vi "Read-all-variables.vi"(8 "error in (no error)":errorcluster, 11 "Config. params. ref. in":refnum<data-value>) -> (0 "error out":errorcluster, 2 "Config. vars.":T1, 3 "Config. params. ref.":refnum<data-value>)   [LabVIEW 2013, in "CameraVision.lvlib" / "CV-Configuration.lvclass"]
uses:
  CV-Configuration.lvclass
  Configuration-variables.ctl
  Hardware/Camera/Camera.lvclass
  UI/Module-states.ctl
  CV-Configuration.lvclass/CV-Configuration.ctl
  UI/CV-UI.lvclass
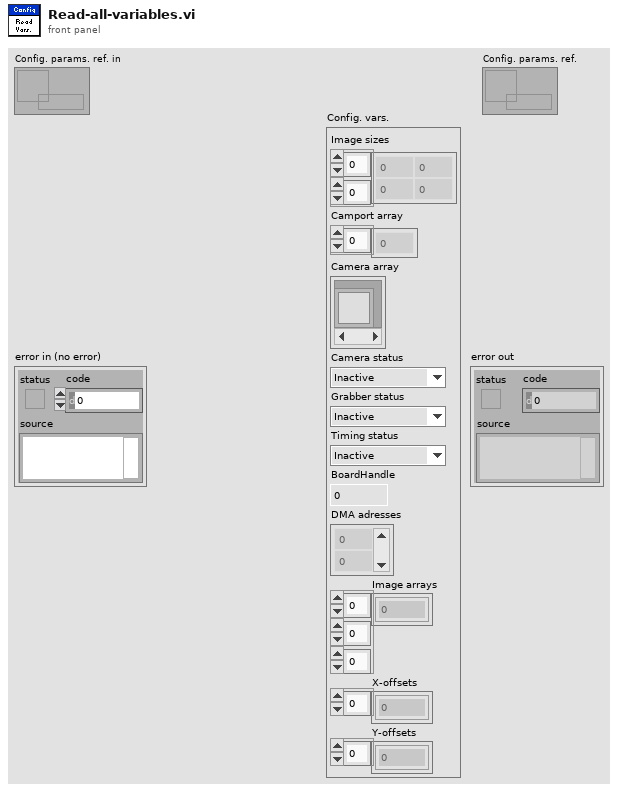
[diagram p1: front panel]
types:
  T1 = typedef "CameraVision.lvlib/CV-Configuration.lvclass/Configuration-variables.ctl" = cluster{"Image sizes":u32[][], "Camport array":u32[], "Camera array":refnum<class "Camera.lvclass">[], "Camera status":T2, "Grabber status":T2, "Timing status":T2, "BoardHandle":u64, "DMA adresses":i64[], "Image arrays":i8[][][], "X-offsets":i32[], "Y-offsets":i32[]}
  T2 = typedef "CameraVision.lvlib/CV-UI.lvclass/Module-states.ctl" = enum16{"Inactive", "Active", "Data-loss", "Error", "Simulation", "Synchronizing", "Initialized", "Released"}
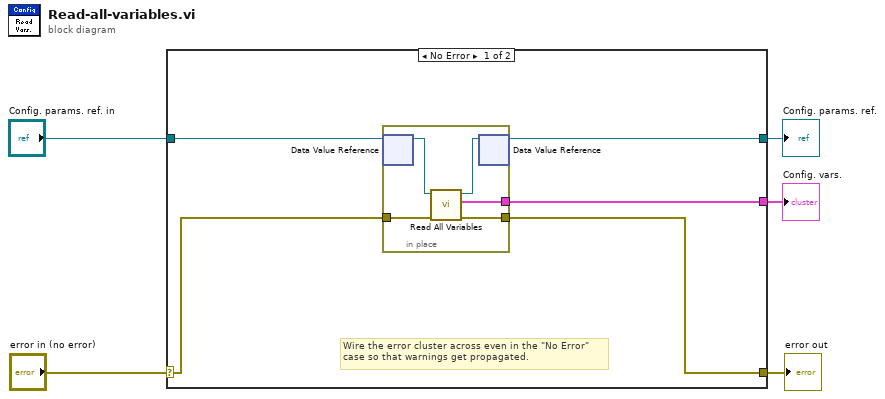
[diagram p0: block diagram]
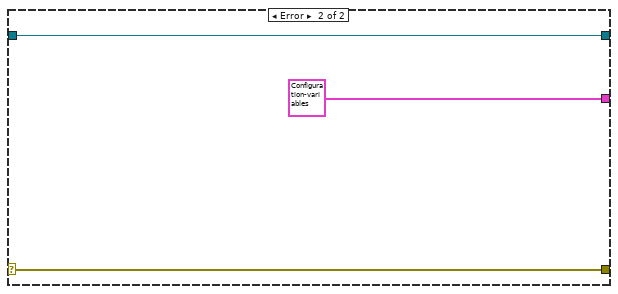
[diagram p2: hidden frame]
diagram:
  n1 = case shown="No Error" "error in (no error)" {
    selector: "error in (no error)" -> [w8 w18]
    tunnel: [w10 w18] -> w4
    tunnel: "Config. params. ref. in" -> [w7 w16]
    tunnel: [w9 T1 {"Image sizes"=[], "Camport array"=[], "Camera array"=[], "Camera status"=enum."Inactive", "Grabber status"=enum."Inactive", "Timing status"=enum."Inactive", "BoardHandle"=0, "DMA adresses"=[], "Image arrays"=[], "X-offsets"=[], "Y-offsets"=[]} ("Config. vars.")] -> w2
    tunnel: [w6 w16] -> w1
    frame No Error {
      # "Wire the error cluster across even in the \"No Error\"\ncase so that warnings get propagated."
      n2 = in-place {
        in-place-border: [w15] -> w10
        in-place-border: [w14] -> w9
        in-place-border: w8 -> [w13]
        n3 = in-place-dvr #1(w7) -> (w11:refnum<class "CV-Configuration.lvclass">)  [unwired: 1 out]
        n4 = call "Read All Variables.vi"("error in (no error)"=w13, "Config params in"=w11) -> ("error out"=w15:errorcluster, "Config. vars."=w14:T1, "Config params out"=w12:refnum<class "CV-Configuration.lvclass">)  [unwired: 7 in]
        n5 = in-place-dvr #1(w12) -> (w6:refnum<data-value>)  [unwired: 1 out]
      }
    }
    frame Error {
    }
  }
  "error out" <- w4
  "Config. params. ref." <- w1
  "Config. vars." <- w2
